vi "Load Impedance.vi"(0 "phase voltage spectra":T2(array[cluster]), 5 "current spectra":T2(array[cluster]), 9 "system info in":refnum<class "EP System Info.lvclass">, 11 "error in (no error)":errorcluster) -> (4 "load impedance":cdb[](array[numeric]), 10 "system info out":refnum<class "EP System Info.lvclass">, 15 "error out":errorcluster)   [LabVIEW 2012, in "NI_EP_Power Quality.lvlib"]
doc: "Calculates the load impedance. You can use the <b>EP D to Y Conversion</b> VI to calculate the <b>phase voltage spectra</b>."
uses:
  <vilib>/addons/Electrical Power/PQ/NI_EP_Power Quality.lvlib
  <vilib>/addons/Electrical Power/PQ/Common/Classes/System Info/EP System Info.lvclass
  <vilib>/addons/Electrical Power/PQ/Common/Controls/ep_AI Data Channel.ctl
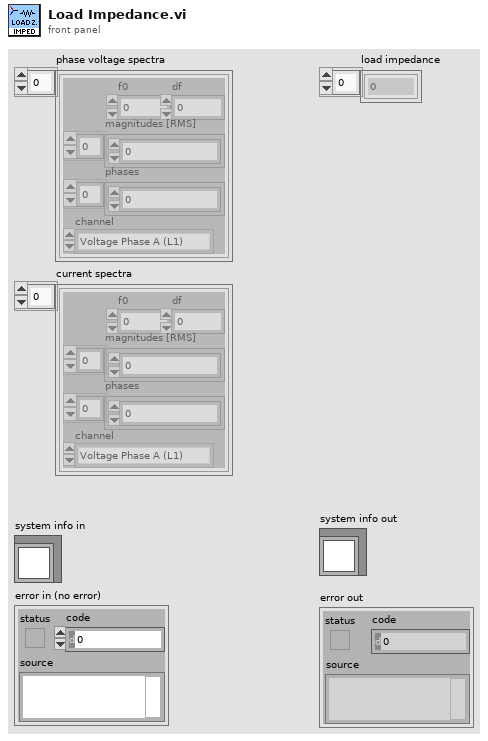
[diagram p1: front panel]
types:
  T1 = typedef "NI_EP_Power Quality.lvlib/ep_AI Data Channel.ctl" = enum16{"Voltage Phase A (L1)", "Voltage Phase B (L2)", "Voltage Phase C (L3)", "Voltage Phase N (Neutral)", "Current Phase A (L1)", "Current Phase B (L2)", "Current Phase C (L3)", "Current Phase N (Neutral)"}
  T2 = cluster{"f0":dbl, "df":dbl, "magnitudes [RMS]":dbl[], "phases":dbl[], "channel":T1}[]
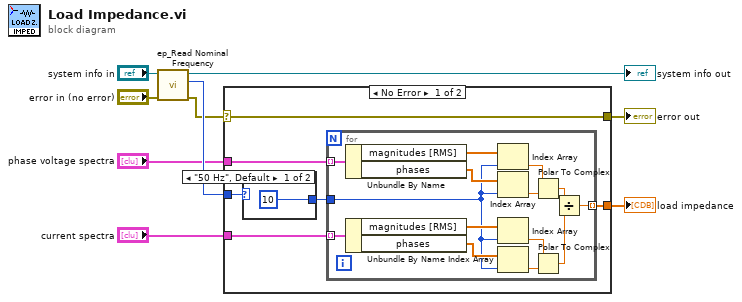
[diagram p0: block diagram]
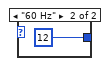
[diagram p2: hidden frame]
diagram:
  n1 = call <vilib>:"ep_Read Nominal Frequency.vi"("error in (no error)"="error in (no error)", "system info in"="system info in") -> ("error out"=w3:errorcluster, "nominal frequency"=w9:enum16{"50 Hz", "60 Hz"}, "system info out"=→"system info out":refnum<class "EP System Info.lvclass">)  [unwired: 6 in, 1 out]
  n2 = case shown="No Error" w3 {
    selector: w3 -> [w10 w32]
    tunnel: "phase voltage spectra" -> [w15 _]
    tunnel: "current spectra" -> [w14 _]
    tunnel: w9 -> [w13 _]
    tunnel: [w11 _] -> w8
    tunnel: [w10 w32] -> w7
    frame No Error {
      n3 = case shown="\"50 Hz\", Default" w13 {
        tunnel: [10 ("index") 12 ("index")] -> w12
        frame "50 Hz", Default {
        }
        frame "60 Hz" {
        }
      }
      n4 = for {
        tunnel: w15 -> [w31] mode=indexing
        tunnel: w14 -> [w30] mode=indexing
        tunnel: w12 -> [w24]
        tunnel: [w29] -> w11 mode=indexing
        n5 = Unbundle By Name(w31) -> ("magnitudes [RMS]"=w28:dbl[], "phases"=w26:dbl[])
        n6 = Unbundle By Name(w30) -> ("magnitudes [RMS]"=w27:dbl[], "phases"=w25:dbl[])
        n7 = Index Array(array=w28, index=w24) -> (element=w23:dbl)
        n8 = Index Array(array=w26, index=w24) -> (element=w22:dbl)
        n9 = Index Array(array=w27, index=w24) -> (element=w20:dbl)
        n10 = Index Array(array=w25, index=w24) -> (element=w19:dbl)
        n11 = Polar To Complex(1:w22, 2:w23) -> (0:w21:cdb)
        n12 = Polar To Complex(1:w19, 2:w20) -> (0:w18:cdb)
        n13 = Divide(x=w21, y=w18) -> (x/y=w29:cdb)
      }
    }
    frame Error {
    }
  }
  "error out" <- w7
  "load impedance" <- w8
